vi "Taiko_TaggedValueListToStrArray.vi"(11 "TaggedValueList":T2 {"Tag" format="%x" items=["NONE"=0, "Locked"=16, "SoftLock"=17, "KeyLock"=18, "Class_IV_Lock"=20, "Interlock"=24, "LaserMode"=32, "LDH_PulsePowerTable"=33, "TriggerMode"=48, "TriggerLevelRaw"=64, "TriggerLevelRawLoLimit"=65, "TriggerLevelRawHiLimit"=66, "TriggerLevel"=72, "TriggerLevelLoLimit"=73, "TriggerLevelHiLimit"=74, "FastGate"=80, "FastGateImp"=96, "SlowGate"=112, "TargetTempRaw"=144, "TargetTempRawLoLimit"=145, "TargetTempRawHiLimit"=146, "CurrentTempRaw"=148, "CaseTempRaw"=149, "TargetTemp"=152, "TargetTempLoLimit"=153, "TargetTempHiLimit"=154, "CurrentTemp"=156, "CaseTemp"=157, "TempScale"=159, "Frequency"=168, "FrequencyLoLimit"=169, "FrequencyHiLimit"=170, "PulsePowerRaw"=176, "PulsePowerRawLoLimit"=177, "PulsePowerRawHiLimit"=178, "PulsePowerPermille"=180, "PulseShape"=181, "PulsePower"=184, "PulsePowerLoLimit"=185, "PulsePowerHiLimit"=186, "PulsePowerNanowatt"=188, "PulsePowerVoltage"=190, "PulseEnergy"=191, "CwPowerRaw"=192, "CwPowerRawLoLimit"=193, "CwPowerRawHiLimit"=194, "CwPowerPermille"=196, "CwPower"=200, "CwPowerLoLimit"=201, "CwPowerHiLimit"=202, "CwPowerMicroWatt"=204, "BurstLen"=208, "BurstPeriod"=224, "LDH_Fan"=240, "UI_Exclusive"=256]}) -> (2 "ValList":string[](array[string]), 3 "TagList":string[](array[string]))   [LabVIEW 2010]
uses:
  _lib/PDLM/pdlm_lib_x86_x64_UIThread.llb/PDLM_Tag.ctl
  _lib/PDLM/pdlm_lib_x86_x64_UIThread.llb/PDLM_TaggedValue.ctl
  _lib/PDLM/pdlm_lib_x86_x64_UIThread.llb/PDLM_TaggedValueList.ctl
  _lib/PDLM/pdlm_lib_x86_x64_UIThread.llb/PDLM_ScaleID.ctl
panel:
  out "ScaleID":T1
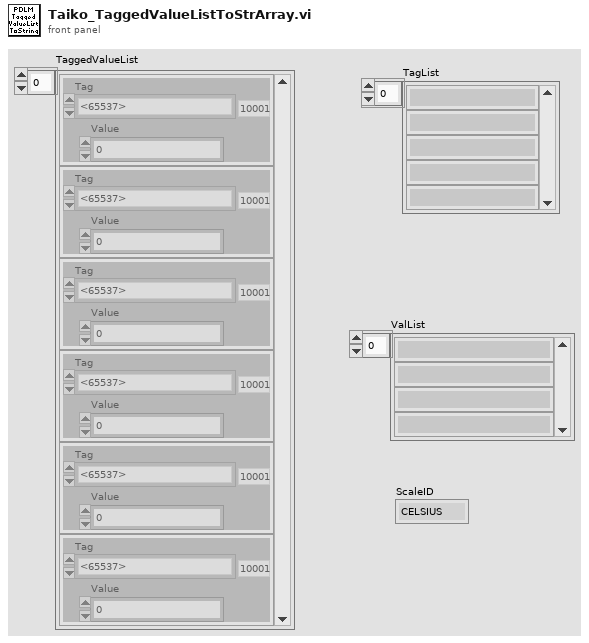
[diagram p1: front panel]
types:
  T1 = typedef "PDLM_ScaleID.ctl" = enum32{"CELSIUS", "FAHRENHEIT", "KELVIN"}
  T2 = typedef "PDLM_TaggedValueList.ctl" = T3[]
  T3 = typedef "PDLM_TaggedValue.ctl" = cluster{"Tag":T4, "Value":u32}
  T4 = typedef "PDLM_Tag.ctl" = u32
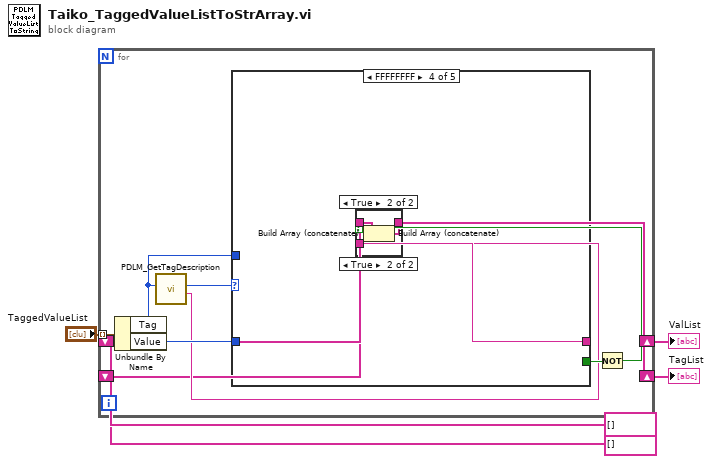
[diagram p0: block diagram]
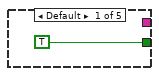
[diagram p4: hidden frame]
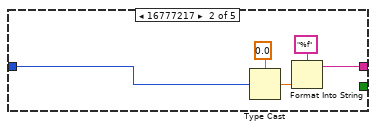
[diagram p5: hidden frame]
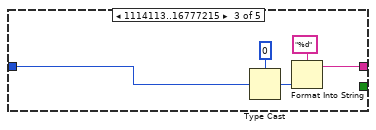
[diagram p6: hidden frame]
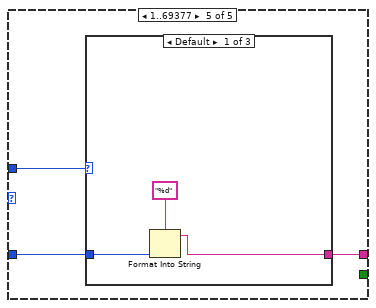
[diagram p7: hidden frame]
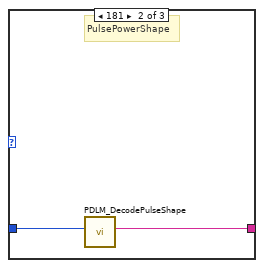
[diagram p8: hidden frame]
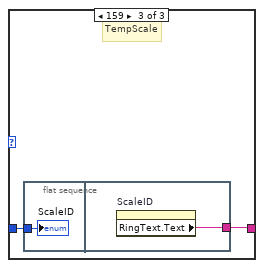
[diagram p9: hidden frame]
diagram:
  n1 = for {
    tunnel: "TaggedValueList" -> [w17] mode=indexing
    shift-right: [w8] -> w4
    shift-left: string[] [] ("Array") -> [w9]
    shift-right: [w6] -> w3
    shift-left: string[] [] ("Array") -> [w7]
    n2 = Unbundle By Name(w17) -> ("Tag"=w10:T4, "Value"=w16:u32)
    n3 = call "PDLM_GetTagDescription.vi"("Tag"=w10) -> ("Name"=w12:string, "TypeCode"=w11:u32)  [unwired: 7 in, 2 out]
    n4 = case shown="FFFFFFFF" w11 {
      tunnel: w16 -> [_ w27 w36 _ w38]
      tunnel: [TRUE _ _ _ _] -> w15
      tunnel: [_ w28 w32 _ w37] -> w14
      tunnel: w10 -> [_ _ _ _ w39]
      frame Default {
      }
      frame 16777217 {
        n5 = Type Cast(type=sgl 0.0, x=w27) -> (*(type *) &x=w30:sgl)
        n6 = Format Into String(format string="%f", w30) -> (resulting string=w28:string)  [unwired: 2 in, 1 out]
      }
      frame 1114113..16777215 {
        n7 = Type Cast(type=0, x=w36) -> (*(type *) &x=w34:i32)
        n8 = Format Into String(format string="%d", w34) -> (resulting string=w32:string)  [unwired: 2 in, 1 out]
      }
      frame -1 {
      }
      frame 1..69377 {
        n9 = case shown="Default" w39 {
          tunnel: w38 -> [w41 w44 w46]
          tunnel: [w40 w43 w45] -> w37
          frame Default {
            n10 = Format Into String(format string="%d", w41) -> (resulting string=w40:string)  [unwired: 2 in, 1 out]
          }
          frame 181 {
            # "PulsePowerShape"
            n11 = call "PDLM_DecodePulseShape.vi"("shape"=w44) -> ("Buffer"=w43:string)  [unwired: 8 in, 2 out]
          }
          frame 159 {
            # "TempScale"
            n12 = flat-sequence {
              tunnel: w46 -> [w47]
              tunnel: [w48] -> w45
              frame #0 {
                "ScaleID" <- w47
              }
              frame #1 {
                n13 = property on="ScaleID" class="Enum (strict)"() -> ("RingText.Text"=w48:string)  [unwired: 2 in, 2 out]
              }
            }
          }
        }
      }
    }
    n14 = Not(x=w15) -> (.not. x?=w13:bool)
    n15 = case shown="True" w13 {
      tunnel: w7 -> [w18 w20]
      tunnel: w12 -> [_ w19]
      tunnel: [w18 w21] -> w6
      frame False {
      }
      frame True {
        n16 = Build Array (concatenate)(w20, w19) -> (w21:string[])
      }
    }
    n17 = case shown="True" w13 {
      tunnel: w9 -> [w22 w24]
      tunnel: w14 -> [_ w23]
      tunnel: [w22 w25] -> w8
      frame False {
      }
      frame True {
        n18 = Build Array (concatenate)(w24, w23) -> (w25:string[])
      }
    }
  }
  "ValList" <- w4
  "TagList" <- w3
